vi "Initialize Output File.vi"(8 "error in (no error)":errorcluster, 11 "File Path Control":path) -> (0 "error out":errorcluster)   [LabVIEW 2017]
uses:
  <vilib>/Utility/file.llb/Write Delimited Spreadsheet (string).vi
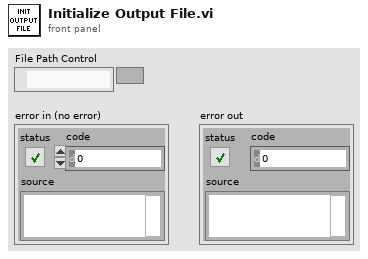
[diagram p1: front panel]
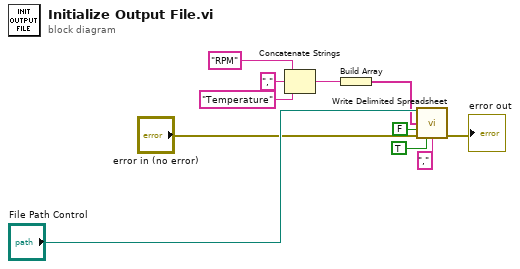
[diagram p0: block diagram]
diagram:
  n1 = Concatenate Strings("RPM" ("string"), "," ("string"), "Temperature" ("string")) -> (w8:string)
  n2 = Build Array(w8) -> (w4:string[])
  n3 = call-poly <vilib>:"Write Delimited Spreadsheet.vi"("file path (dialog if empty)"="File Path Control", "1D data"=w4, "append to file? (new file:F)"=FALSE, "error in (no error)"="error in (no error)", "transpose? (no:F)"=TRUE, "delimiter (\\t)"="," ("delimiter (\\t)")) -> ("error out"=→"error out":errorcluster)  [unwired: 8 in, 1 out]
